vi "高锰酸钾-ORP滴定曲线(子VI).vi"   [LabVIEW 2016, in "斯坦道CODMn新电路板.lvlib"]
uses:
  <vilib>/ptbypt/NI_PtbyPt.lvlib
types:
  T1 = enum16{"空闲", "水样测试", "标样核查", "零点核查", "跨度核查", "空白测试", "平行样测试", "加标回收", "空白校准", "标样校准", "初始化（清洗）"}
  T2 = cluster{"系统时间":timestamp, "工作状态":u16, "测量模式":enum16{"待机", "连续模式", "周期模式", "定点模式", "受控模式", "手动模式"}, "告警代码":u16, "故障代码":u16, "日志代码":u16, "软件版本":u16, "A":sgl, "B":sgl, "K":sgl, "当前滴定数":sgl, "T":sgl, "H":sgl, "id":u16, "flowid":u16, "量程":u16, "加热实时温度":sgl, "当前ORP值":sgl, "运行时间":sgl, "当前步骤剩余时间":sgl, "结束滴定数":sgl, "注射泵保温温度":sgl}
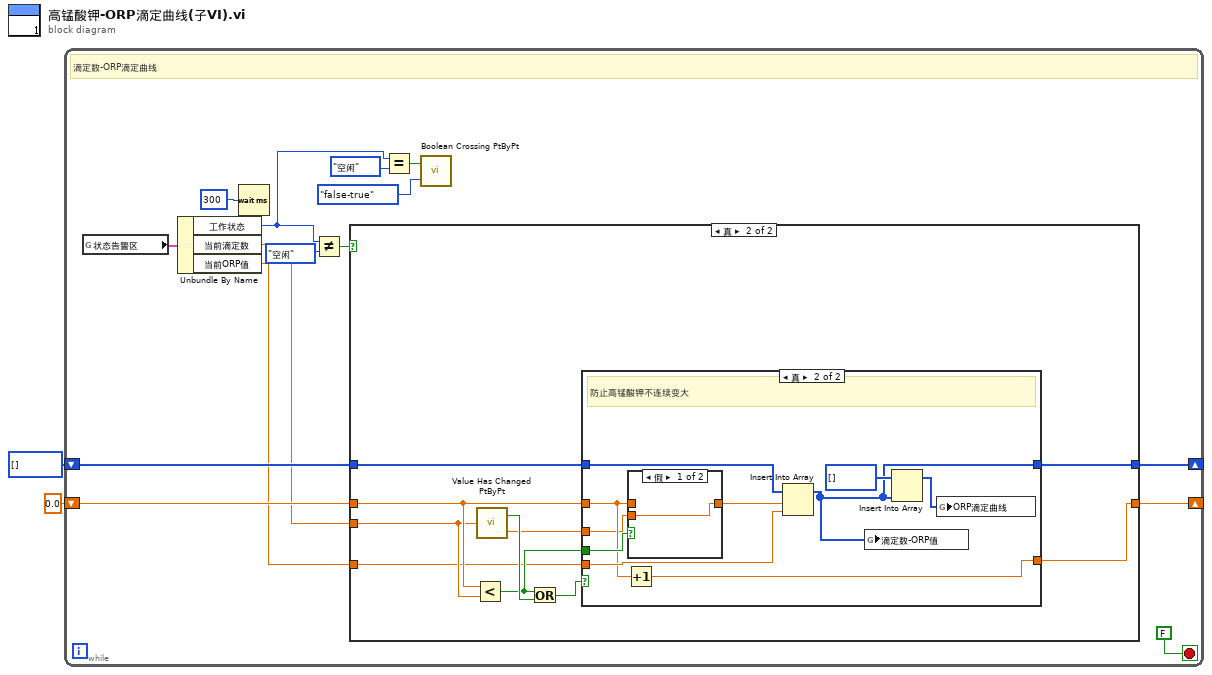
[diagram p0: block diagram]
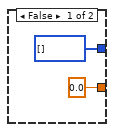
[diagram p2: hidden frame]
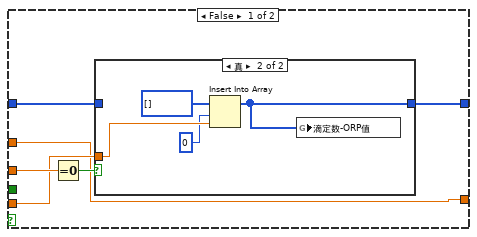
[diagram p3: hidden frame]
diagram:
  n1 = while {
    shift-right: [w14] -> _
    shift-left: u16[] [] ("ORP滴定曲线") -> [w15]
    shift-right: [w12] -> _
    shift-left: 0.0 -> [w13]
    stop <- FALSE stop-if-true
    # "滴定数-ORP滴定曲线"
    n2 = global read "VARCODMn全局变量.vi" "状态告警区"() -> (w11:T2)
    n3 = Unbundle By Name(w11) -> ("工作状态"=w3:u16, "当前滴定数"=w8:sgl, "当前ORP值"=w7:sgl)
    n4 = Wait (ms)(milliseconds to wait=u32 300 ("等待时间（毫秒）")) -> ()  [unwired: 1 out]
    n5 = Not Equal?(x=w3, y=T1."空闲" ("工作状态")) -> (x != y?=w9:bool)
    n6 = case shown="真" w9 {
      tunnel: w15 -> [_ w29]
      tunnel: [u16[] [] ("ORP滴定曲线") w28] -> w14
      tunnel: w13 -> [_ w24]
      tunnel: [0.0 w23] -> w12
      tunnel: w8 -> [_ w21]
      tunnel: w7 -> [_ w20]
      frame False {
      }
      frame True {
        n7 = Less?(x=w24, y=w21) -> (x < y?=w22:bool)
        n8 = call <vilib>:"Value Has Changed PtByPt.vi"("input data point"=w21) -> ("has changed"=w27:bool, "output data point"=w26:dbl)  [unwired: 1 in]
        n9 = Or(x=w22, y=w27) -> (x .or. y?=w25:bool)
        n10 = case shown="真" w25 {
          tunnel: w29 -> [w34 w49]
          tunnel: [w33 w41] -> w28
          tunnel: w26 -> [w35 w43]
          tunnel: w20 -> [w31 w48]
          tunnel: w24 -> [w30 w45]
          tunnel: [w30 w47] -> w23
          tunnel: w22 -> [_ w46]
          frame False {
            n11 = Equal To 0?(x=w35) -> (x = 0?=w32:bool)
            n12 = case shown="真" w32 {
              tunnel: [w36 w37] -> w33
              tunnel: w34 -> [w36 _]
              tunnel: w31 -> [_ w39]
              frame False {
              }
              frame True {
                n13 = Insert Into Array(array=u16[] [] ("ORP滴定曲线"), index=0 ("索引"), new element=w39) -> (w37:u16[])
                n14 = global write "VARCODMn全局变量.vi" "滴定数-ORP值"(w37) -> ()
              }
            }
          }
          frame True {
            # "防止高锰酸钾不连续变大"
            n15 = Increment(x=w45) -> (x+1=w47:dbl)
            n16 = case shown="假" w46 {
              tunnel: w45 -> [_ w52]
              tunnel: [w51 w52] -> w44
              tunnel: w43 -> [w51 _]
              frame False {
              }
              frame True {
              }
            }
            n17 = Insert Into Array(array=w49, index=w44, new element=w48) -> (w41:u16[])
            n18 = global write "VARCODMn全局变量.vi" "滴定数-ORP值"(w41) -> ()
            n19 = Insert Into Array(array=u16[] [] ("ORP滴定曲线"), new element=w41) -> (w42:u16[])  [unwired: 1 in]
            n20 = global write "VARCODMn全局变量.vi" "ORP滴定曲线"(w42) -> ()
          }
        }
      }
    }
    n21 = Equal?(x=w3, y=T1."空闲" ("工作状态")) -> (x = y?=w5:bool)
    n22 = call <vilib>:"Boolean Crossing PtByPt.vi"("direction"=enum16{"either", "false-true", "true-false"}."false-true", "input"=w5) -> ()  [unwired: 1 in, 1 out]
  }
